vi "find_surface_simple2.vi"(8 "error in":errorcluster, 9 "Struc El Size":i32=10, 10 "Threshold Multiplier":sgl=2.0, 11 "Image In":T1=refnum) -> (0 "error out":errorcluster, 3 "average surface height":dbl=-1.0 format="%0.2f")   [LabVIEW 2016]
doc: "Estimates position of top surface of B-scan. Use thresholding to binarise image, morphological operations to remove holes and islands, and then find first '1' along each column. Returns vector of\nheights for each column and median value. Median does not include '0' surface \nheight detections which usually correspond to an artefact."
uses:
  <vilib>/vision/Image Controls.llb/IMAQ Image.ctl
  <vilib>/vision/NI_Vision_Development_Module.lvlib
  <vilib>/Analysis/NI_AALBase.lvlib
panel:
  out "surface heights":i32[](array[numeric])=[-1, -1, -1, -1, -1, -1, -1, -1, -1, -1, -1, -1, -1, -1, -1, -1, -1, -1, -1, -1, -1, -1, -1, -1, -1, -1, -1, -1, -1, -1, -1, -1, -1, -1, -1, -1, -1, -1, -1, -1, -1, -1, -1, -1, -1, -1, -1, -1, -1, -1, -1, -1, -1, -1, -1, -1, -1, -1, -1, -1, -1, -1, -1, -1, -1, -1, -1, -1, -1, -1, -1, -1, -1, -1, -1, -1, -1, -1, -1, -1, -1, -1, -1, -1, -1, -1, -1, -1, -1, -1, -1, -1, -1, -1, -1, -1, -1, -1, -1, -1, -1, -1, -1, -1, -1, -1, -1, -1, -1, -1, -1, -1, -1, -1, -1, -1, -1, -1, -1, -1, -1, -1, -1, -1, -1, -1, -1, -1, -1, -1, -1, -1, -1, -1, -1, -1, -1, -1, -1, -1, -1, -1, -1, -1, -1, -1, -1, -1, -1, -1, -1, -1, -1, -1, -1, -1, -1, -1, -1, -1, -1, -1, -1, -1, -1, -1, -1, -1, -1, -1, -1, -1, -1, -1, -1, -1, -1, -1, -1, -1, -1, -1, -1, -1, -1, -1, -1, -1, -1, -1, -1, -1, -1, -1, -1, -1, -1, -1, -1, -1]
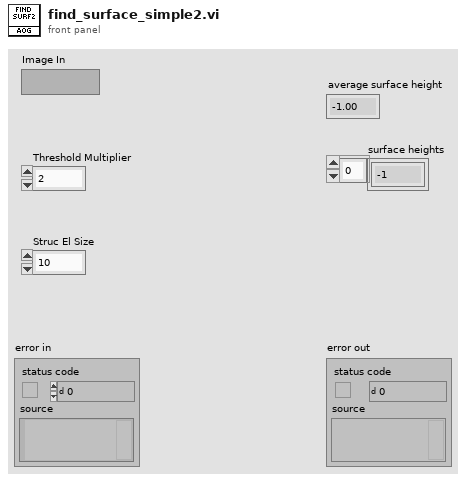
[diagram p1: front panel]
types:
  T1 = typedef "IMAQ Image.ctl" = refnum<image>
  T2 = enum32{"AutoM", "Close", "Dilate", "Erode", "Gradient", "Gradient out", "Gradient in", "Hit miss", "Open", "PClose", "POpen", "Thick", "Thin"}
  T3 = cluster{"histogram":u32[], "Minimal Value":sgl, "Maximal Value":sgl, "Starting Value":sgl, "Interval Width":sgl, "Mean Value":sgl, "Standard  Variation":sgl, "Area (pixels)":i32}
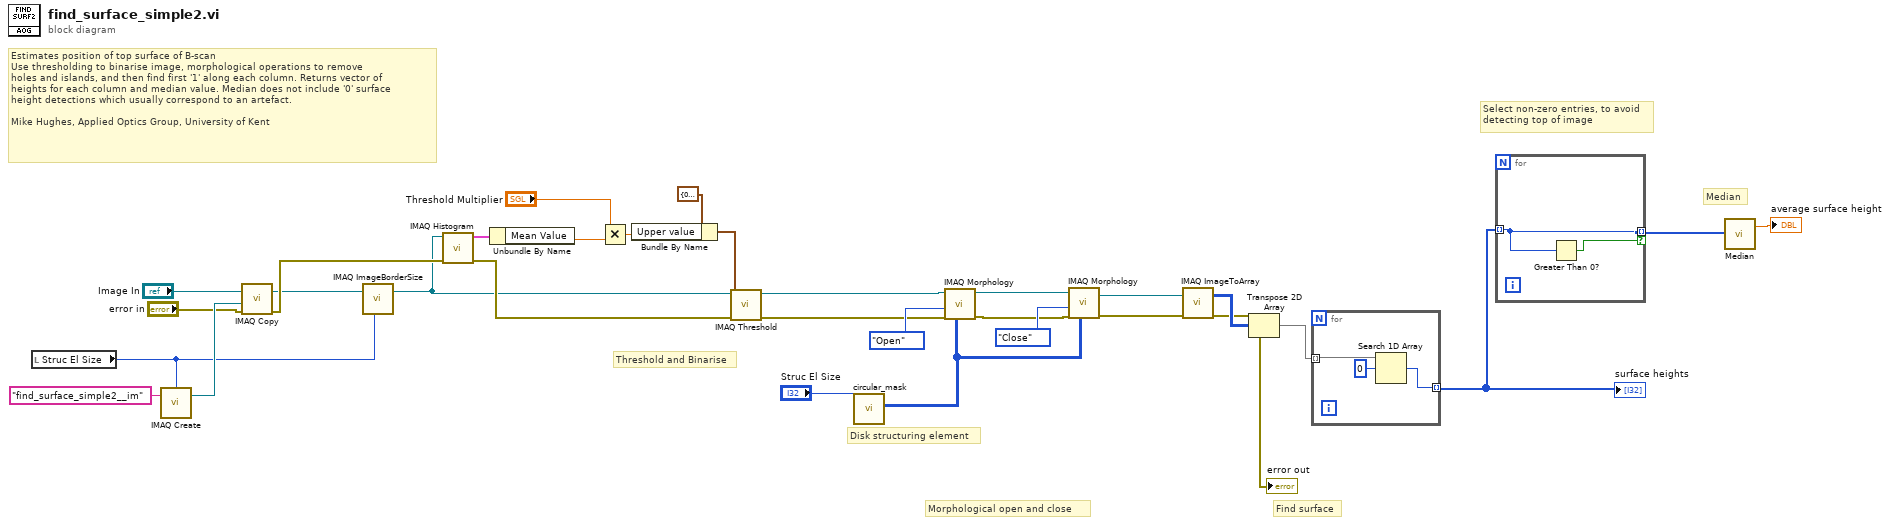
[diagram p0: block diagram]
diagram:
  # "Select non-zero entries, to avoid\ndetecting top of image"
  # "Median"
  # "Disk structuring element"
  # "Find surface"
  # "Morphological open and close"
  # "Threshold and Binarise"
  # "Estimates position of top surface of B-scan\nUse thresholding to binarise image, morphological operations to remove\nholes and islands, and then find first '1' along each column. Returns vector of\nheights for each column and median value. Median does not include '0' surface \nheight detections which usually correspond to an artefact.\n\nMike Hughes, Applied Optics Group, University of Kent"
  n1 = local read "Struc El Size"() -> (w3:i32)
  n2 = call "IMAQ Create"("Border Size"=w3, "Image Name"="find_surface_simple2__im") -> ("New Image"=w15:T1)  [unwired: 3 in, 1 out]
  n3 = call "IMAQ Copy"("error in (no error)"="error in", "Image Dst"=w15, "Image Src"="Image In") -> ("error out"=w13:errorcluster, "Image Dst Out"=w5:T1)  [unwired: 3 in]
  n4 = call "IMAQ ImageBorderSize"("Image"=w5, "Image border size in"=w3) -> ("Image Out"=w4:T1)  [unwired: 2 in, 2 out]
  n5 = call "IMAQ Histogram"("error in (no error)"=w13, "Image"=w4) -> ("error out"=w17:errorcluster, "Histogram Report"=w31:T3)  [unwired: 8 in]
  n6 = Unbundle By Name(w31) -> ("Mean Value"=w30:sgl)
  n7 = Multiply(x="Threshold Multiplier", y=w30) -> (x*y=w27:sgl)
  n8 = Bundle By Name(cluster=cluster{"Lower value":sgl, "Upper value":sgl} {"Lower value"=0.0, "Upper value"=255.0} ("Range"), "Upper value"=w27) -> (w26:cluster{"Lower value":sgl, "Upper value":sgl})
  n9 = call "IMAQ Threshold"("error in (no error)"=w17, "Range"=w26, "Image Src"=w4) -> ("error out"=w11:errorcluster, "Image Dst Out"=w22:T1)  [unwired: 7 in]
  n10 = call "circular_mask.vi"("size"="Struc El Size") -> ("Mask Array"=w6:i16[][])  [unwired: 10 in]
  n11 = call "IMAQ Morphology"("Structuring Element"=w6, "error in (no error)"=w11, "Operation"=T2."Open", "Image Src"=w22) -> ("error out"=w10:errorcluster, "Image Dst Out"=w24:T1)  [unwired: 6 in]
  n12 = call "IMAQ Morphology"("Structuring Element"=w6, "error in (no error)"=w10, "Operation"=T2."Close", "Image Src"=w24) -> ("error out"=w9:errorcluster, "Image Dst Out"=w21:T1)  [unwired: 6 in]
  n13 = call "IMAQ ImageToArray"("error in (no error)"=w9, "Image"=w21) -> ("error out"=→"error out":errorcluster, "Image Pixels (U8)"=w20:u8[][])  [unwired: 2 in, 3 out]
  n14 = Transpose 2D Array(2D array=w20) -> (transposed array=w19:u8[][])
  n15 = for {
    tunnel: w19 -> [w34] mode=indexing
    tunnel: [w32] -> w2 mode=indexing
    n16 = Search 1D Array(1D array=w34, element=u8 0) -> (index of element=w32:i32)  [unwired: 1 in]
  }
  "surface heights" <- w2
  n17 = for {
    tunnel: w2 -> [w36] mode=indexing
    tunnel: [w36] -> w1 mode=indexing if=w35
    n18 = Greater Than 0?(x=w36) -> (x > 0?=w35:bool)
  }
  n19 = call <vilib>:"Median.vi"("X"=w1) -> ("median"=→"average surface height":dbl)  [unwired: 1 out]
